vi "Analog Set Reference Voltage.vi"(8 "Error In":errorcluster, 9 "Analog Reference (V)":dbl=5.0, 10 "AI Reference Mode":T7=enum."Internal", 11 "LINX Ref in":T1) -> (0 "Error Out":errorcluster, 3 "LINX Ref out":T1)   [LabVIEW 2014, in "LMH-LINX.lvlib"]
doc: "Set the analog input reference voltage. Supported modes (internal/external) and values depend on the LINX device."
uses:
  LMH-LINX.lvlib
  Private/Device/Type Defs/AI Reference Mode.ctl
  Private/Type Defs/LINX Ref.ctl
  Private/Type Defs/Platform.ctl
  Private/Type Defs/Interface.ctl
  Private/Device/Type Defs/LINX Device Config.ctl
  Private/Device/Type Defs/TCP Config.ctl
  Private/Device/Type Defs/Channels.ctl
  Private/Type Defs/Error Type.ctl
  Private/Device/Device.lvlib
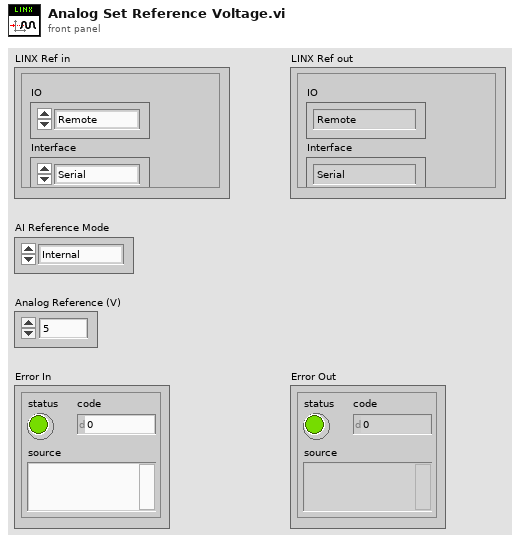
[diagram p1: front panel]
types:
  T1 = typedef "LMH-LINX.lvlib/LINX Ref.ctl" = cluster{"IO":T2, "Interface":T3, "LINX Device Config":T4}
  T2 = typedef "LMH-LINX.lvlib/Platform.ctl" = enum16{"Remote", "Local"}
  T3 = typedef "LMH-LINX.lvlib/Interface.ctl" = enum16{"Serial", "TCP"}
  T4 = typedef "LMH-LINX.lvlib/Device.lvlib/LINX Device Config.ctl" = cluster{"Interface":T3, "COM Port":refnum<visa-resource-name>, "TCP Configuration":T5, "Device Family":u8, "Device ID":u8, "Device Name":string, "TCP Ref":refnum<k5>, "Channels":T6}
  T5 = typedef "LMH-LINX.lvlib/Device.lvlib/TCP Config.ctl" = cluster{"IP Address":string, "Port":u16}
  T6 = typedef "LMH-LINX.lvlib/Channels.ctl" = cluster{"DI":u8[], "DO":u8[], "AI":u8[], "AO":u8[], "PWM":u8[], "QE":u8[], "UART":u8[], "I2C 2":u8[], "SPI":u8[], "CAN":u8[], "Servo":u8[], "AI Ref (V)":dbl, "AO Ref (V)":dbl, "AO Resolution (Bits)":u8}
  T7 = typedef "LMH-LINX.lvlib/Device.lvlib/AI Reference Mode.ctl" = enum16{"Default", "Internal", "External"}
  T8 = typedef "LMH-LINX.lvlib/Error Type.ctl" = enum16{"Unknown", "Timeout", "Corrupt Return Packet", "Unable To Connect", "Command Not Supported", "Channel DNE", "Invalid COM Config", "Firmware Version Mismatch", "myRIO Support", "CMD Specific Error"}
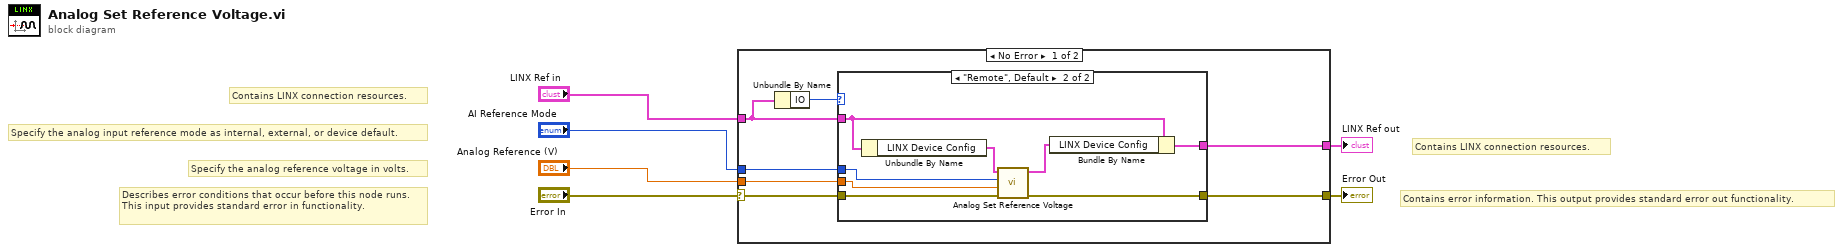
[diagram p0: block diagram]
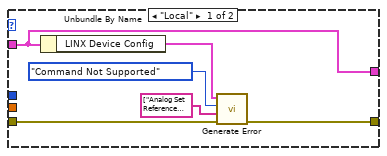
[diagram p2: hidden frame]
diagram:
  # "Specify the analog reference voltage in volts."
  # "Specify the analog input reference mode as internal, external, or device default."
  # "Contains LINX connection resources."
  # "Contains error information. This output provides standard error out functionality."
  # "Contains LINX connection resources."
  # "Describes error conditions that occur before this node runs. This input provides standard error in functionality."
  n1 = case shown="No Error" "Error In" {
    selector: "Error In" -> [w9 w28]
    tunnel: "Analog Reference (V)" -> [w13 _]
    tunnel: "AI Reference Mode" -> [w12 _]
    tunnel: [w11 w29] -> w5
    tunnel: [w10 w28] -> w4
    tunnel: "LINX Ref in" -> [w7 w29]
    frame No Error {
      n2 = Unbundle By Name(w7) -> ("IO"=w8:T2)
      n3 = case shown="\"Remote\", Default" w8 {
        tunnel: w13 -> [_ w22]
        tunnel: w12 -> [_ w23]
        tunnel: [w14 w27] -> w11
        tunnel: [w19 w20] -> w10
        tunnel: w7 -> [w14 w26]
        tunnel: w9 -> [w18 w21]
        frame "Local" {
          n4 = Unbundle By Name(w14) -> ("LINX Device Config"=w17:T4)
          n5 = call "Generate Error.vi"("Error In"=w18, "Arguments"=string[] ["Analog Set Reference Voltage"], "Error Type"=Error_Type."Command Not Supported", "LINX Device Config"=w17) -> ("Error Out"=w19:errorcluster)  [unwired: 6 in, 1 out]
        }
        frame "Remote", Default {
          n6 = Unbundle By Name(w26) -> ("LINX Device Config"=w24:T4)
          n7 = call "Analog Set Reference Voltage.vi"("Error In"=w21, "Voltage (V)"=w22, "Analog Reference Mode"=w23, "LINX Device Config"=w24) -> ("Error Out"=w20:errorcluster, "LINX Device Config"=w25:T4)  [unwired: 6 in]
          n8 = Bundle By Name(cluster=w26, "LINX Device Config"=w25) -> (w27:T1)
        }
      }
    }
    frame Error {
    }
  }
  "LINX Ref out" <- w5
  "Error Out" <- w4
